vi "Roll Pitch Yaw.vi"(1 "Transformation matrix":T1) -> (0 "Euler Angles":cluster{"roll":dbl, "pitch":dbl, "yaw":dbl})   [LabVIEW 2024]
uses:
  <vilib>/Analysis/Matrix/Datatypes/RealMatrix.ctl
  <vilib>/Analysis/coordinate.llb/Euler Rotation Order.ctl
  <vilib>/Analysis/NI_AALPro.lvlib
  <vilib>/Analysis/Matrix/NI_Matrix.lvlib
panel:
  out "Euler Angles":cluster{"phi":dbl, "theta":dbl, "psi":dbl}
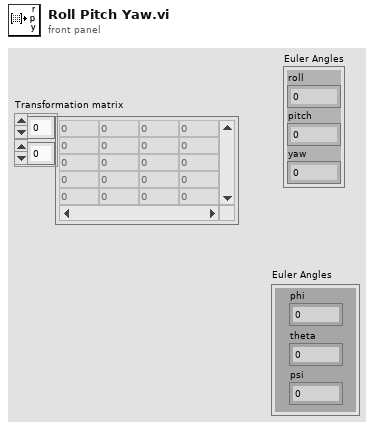
[diagram p1: front panel]
types:
  T1 = typedef "NI_Matrix.lvlib/RealMatrix.ctl" = dbl[][]
  T2 = typedef "NI_AALPro.lvlib/Euler Rotation Order.ctl" = u16
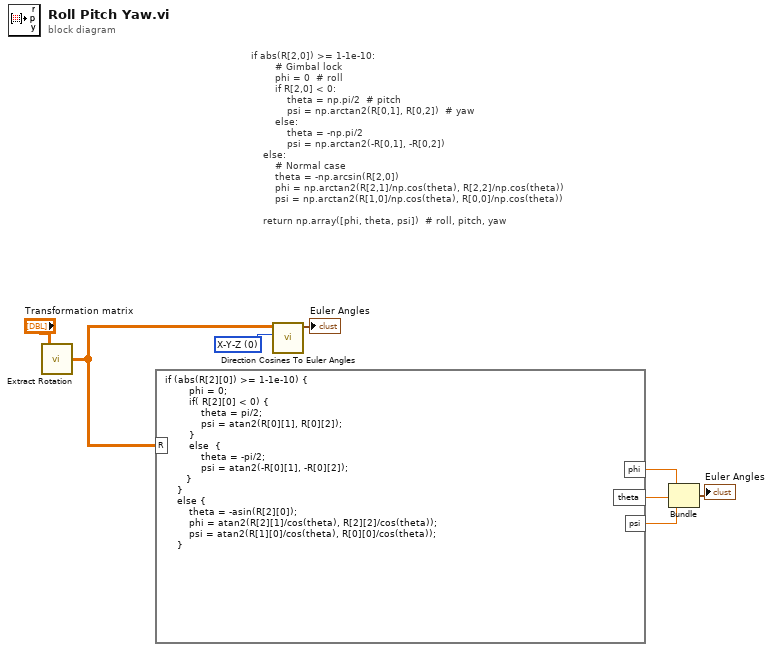
[diagram p0: block diagram]
diagram:
  w8 = T2 0 items=["X-Y-Z", "X-Z-Y", "Y-X-Z", "Y-Z-X", "Z-X-Y", "Z-Y-X", "X-Y-X", "X-Z-X", "Y-X-Y", "Y-Z-Y", "Z-X-Z", "Z-Y-Z"] ("rotation order")
  # "if abs(R[2,0]) >= 1-1e-10:\n        # Gimbal lock\n        phi = 0  # roll\n        if R[2,0] < 0:\n            theta = np.pi/2  # pitch\n            psi = np.arctan2(R[0,1], R[0,2])  # yaw\n        else:\n            theta = -np.pi/2\n            psi = np.arctan2(-R[0,1], -R[0,2])\n    else:\n        # Normal case\n        theta = -np.arcsin(R[2,0])\n        phi = np.arctan2(R[2,1]/np.cos(theta), R[2,2]/np.cos(theta))\n        psi = np.arctan2(R[1,0]/np.cos(theta), R[0,0]/np.cos(theta))\n    \n    return np.array([phi, theta, psi])  # roll, pitch, yaw"
  n1 = call <userlib>:"Extract Rotation.vi"("Transformation matrix"="Transformation matrix") -> ("Rotation matrix"=w1:T1)
  n2 = formula code="if (abs(R[2][0]) >= 1-1e-10) {\n        phi = 0;  \n        if( R[2][0] < 0) {\n            theta = pi/2;\n            psi = atan2(R[0][1], R[0][2]); \n        }\n        else  {\n            theta = -pi/2;\n            psi = atan2(-R[0][1], -R[0][2]);\n       }\n    }\n    else {\n        theta = -asin(R[2][0]);\n        phi = atan2(R[2][1]/cos(theta), R[2][2]/cos(theta));\n        psi = atan2(R[1][0]/cos(theta), R[0][0]/cos(theta));\n    }"("R"=w1) -> ("phi"=w7:dbl, "theta"=w6:dbl, "psi"=w5:dbl)
  n3 = call <vilib>:"Direction Cosines To Euler Angles.vi"("rotation order"=w8, "Direction Cosines"=w1) -> ("Euler Angles"=→"Euler Angles":cluster{"phi":dbl, "theta":dbl, "psi":dbl})  [unwired: 8 in, 1 out]
  n4 = Bundle("phi"=w7, "theta"=w6, "psi"=w5) -> (→"Euler Angles":cluster{"phi":dbl, "theta":dbl, "psi":dbl})  [unwired: 1 in]
